vi "Utility folder.vi"(8 "error in (no error)":errorcluster, 9 "Action":T1) -> (0 "error out":errorcluster, 1 "Output":string)   [LabVIEW 2015]
doc: "Constants, which are necessary for the virtual folder <B>Utility</B> in the generated custom device project."
uses:
  Constants TypDef/Utility folder.ctl
  Constants TypDef/Common.ctl
  Common.vi
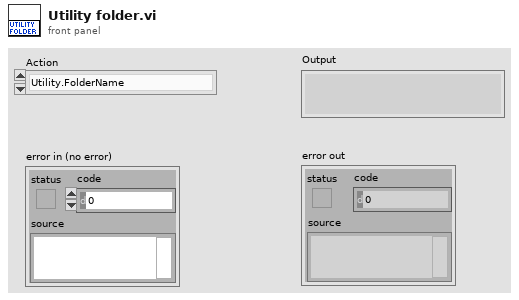
[diagram p1: front panel]
types:
  T1 = typedef "Utility folder.ctl" = enum16{"Utility.FolderName", "Utility.Copy .llb to NI VeriStand dir.FileName", "Utility.Copy .llb to NI VeriStand dir.FilePathAndName", "Utility.LLB Pre Build.FilePathAndName"}
  T2 = typedef "Common.ctl" = enum16{"ProjectName", "TemplatesFolderName", "ProjectTemplatePathAndName", "ReadmeTemplatePathAndName", "TimingAndSyncFolderName", "CustomDeviceFolderName", "PathToTemplates"}
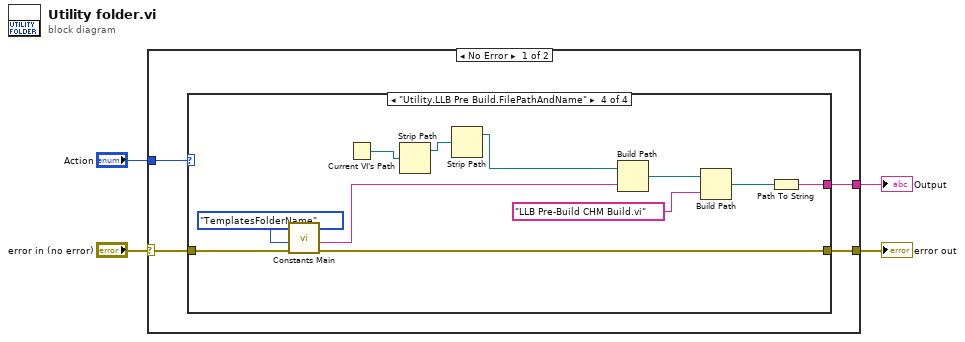
[diagram p0: block diagram]
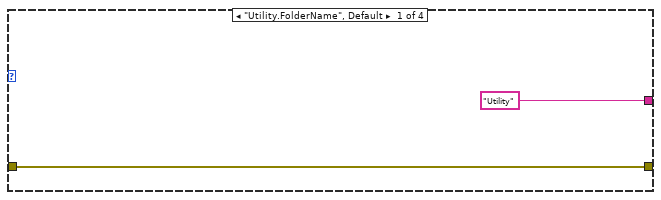
[diagram p2: hidden frame]
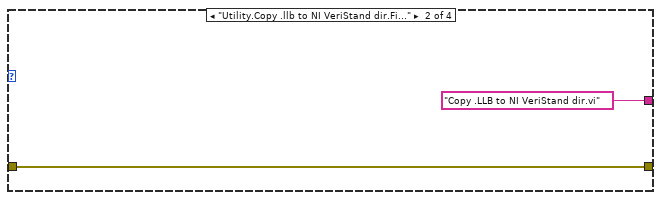
[diagram p3: hidden frame]
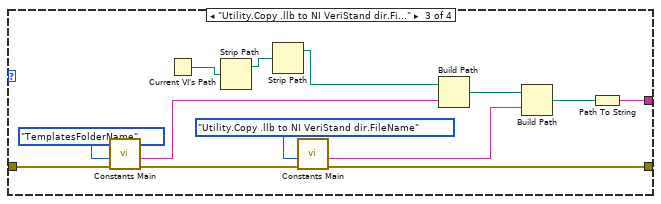
[diagram p4: hidden frame]
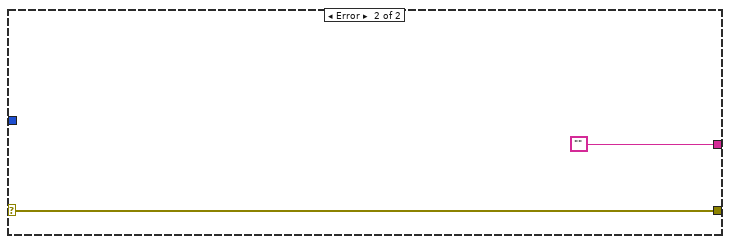
[diagram p5: hidden frame]
diagram:
  n1 = case shown="No Error" "error in (no error)" {
    selector: "error in (no error)" -> [w6 w38]
    tunnel: [w5 w38] -> w2
    tunnel: [w7 ""] -> w1
    tunnel: "Action" -> [w8 _]
    frame No Error {
      n2 = case shown="\"Utility.LLB Pre Build.FilePathAndName\"" w8 {
        tunnel: ["Utility" "Copy .LLB to NI VeriStand dir.vi" ("name or relative path") w21 w32] -> w7
        tunnel: w6 -> [w9 w11 w22 w33]
        tunnel: [w9 w11 w18 w30] -> w5
        frame "Utility.FolderName", Default {
        }
        frame "Utility.Copy .llb to NI VeriStand dir.FileName" {
        }
        frame "Utility.Copy .llb to NI VeriStand dir.FilePathAndName" {
          n3 = call-poly "Constants Main.vi"("error in (no error)"=w22, "Action"=Common."TemplatesFolderName") -> ("error out"=w19:errorcluster, "Output"=w25:string)  [unwired: 8 in]
          n4 = Current VI's Path() -> (path=w15:path)
          n5 = Strip Path(path=w15) -> (stripped path=w14:path)  [unwired: 1 out]
          n6 = Strip Path(path=w14) -> (stripped path=w13:path)  [unwired: 1 out]
          n7 = call-poly "Constants Main.vi"("error in (no error)"=w19, "Action"=Utility_folder."Utility.Copy .llb to NI VeriStand dir.FileName") -> ("error out"=w18:errorcluster, "Output"=w16:string)  [unwired: 8 in]
          n8 = Build Path(base path=w13, name or relative path=w25) -> (appended path=w24:path)
          n9 = Build Path(base path=w24, name or relative path=w16) -> (appended path=w20:path)
          n10 = Path To String(path=w20) -> (string=w21:string)
        }
        frame "Utility.LLB Pre Build.FilePathAndName" {
          n11 = call-poly "Constants Main.vi"("error in (no error)"=w33, "Action"=Common."TemplatesFolderName") -> ("error out"=w30:errorcluster, "Output"=w36:string)  [unwired: 8 in]
          n12 = Current VI's Path() -> (path=w29:path)
          n13 = Strip Path(path=w29) -> (stripped path=w28:path)  [unwired: 1 out]
          n14 = Strip Path(path=w28) -> (stripped path=w27:path)  [unwired: 1 out]
          n15 = Build Path(base path=w27, name or relative path=w36) -> (appended path=w35:path)
          n16 = Build Path(base path=w35, name or relative path="LLB Pre-Build CHM Build.vi") -> (appended path=w31:path)
          n17 = Path To String(path=w31) -> (string=w32:string)
        }
      }
    }
    frame Error {
    }
  }
  "error out" <- w2
  "Output" <- w1
